vi "CRYFlatten Text Save.vi"(5 "Origin Text":string, 6 "error in":errorcluster, 7 "Type In":enum16{"Curves", "Values", "Results", "WFM"}(ring), 8 "Any Flatten Data":string, 9 "Path In":path) -> (0 "error out":errorcluster, 3 "Path Out":path)   [LabVIEW 2013]
uses:
  CRYSystem/Typedef Control/CRYData Cluster Array.ctl
  CRYSystem/Typedef Control/CRYData Cluster.ctl
  CRYSystem/Typedef Control/CRYWaveform Cluster Array.ctl
  CRYSystem/Typedef Control/CRYWaveform Cluster.ctl
  CRYSystem/Typedef Control/CRYResult Cluster Array.ctl
  CRYSystem/Typedef Control/CRYResult Cluster.ctl
panel:
  in  "Results":T1 {"Margin" format="%.2f"}
  in  "Waveforms":T3 {"Y dB ref" format="%.1f"; "Y axis" items=["Log", "Lin"]; "Y data" items=["dB", "Lin"]; "X data" items=["dB", "Lin"]}
  in  "Curves":T5 {"Z data" items=["dB", "Lin"]; "X data" items=["dB", "Lin"]; "Y data" items=["dB", "Lin"]; "Z dB ref" format="%.1f"; "Z axis" items=["Log", "Lin"]; "X dB ref" format="%.1f"; "X axis" items=["Log", "Lin"]; "Y axis" items=["Log", "Lin"]; "Y dB ref" format="%.1f"; "Curve"."z" format="%.2f"; "Curve"."y" format="%.2f"; "Curve"."x" format="%.2f"}
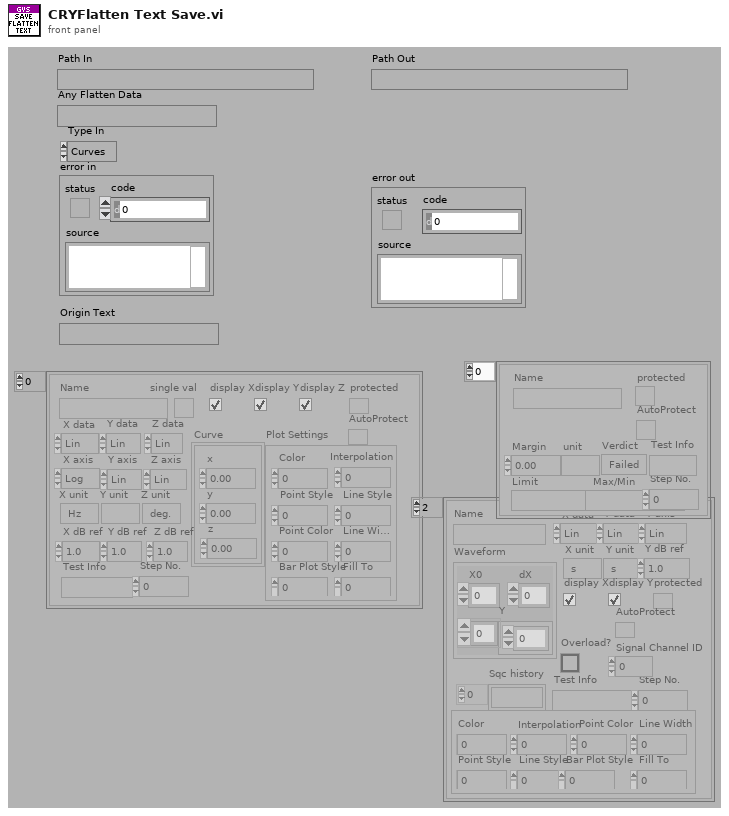
[diagram p1: front panel]
types:
  T1 = typedef "CRYResult Cluster Array.ctl" = T2[]
  T2 = typedef "CRYResult Cluster.ctl" = cluster{"Name":string, "Margin":dbl, "unit":string, "Verdict":bool, "Limit":string, "Max/Min":string, "protected":bool, "Step No.":i32, "Test Info":string, "AutoProtect":bool}
  T3 = typedef "CRYWaveform Cluster Array.ctl" = T4[]
  T4 = typedef "CRYWaveform Cluster.ctl" = cluster{"Waveform":cluster{"X0":dbl, "dX":dbl, "Y":sgl[]}, "X data":u16, "Y data":u16, "Y axis":u16, "X unit":string, "Y unit":string, "Y dB ref":dbl, "display Y":bool, "display X":bool, "Overload?":bool, "Test Info":string, "Step No.":i32, "Name":string, "protected":bool, "Sqc history":string[], "Signal Channel ID":i32, "Plot Settings":cluster{"Color":u32, "Interpolation":u8, "Point Style":u8, "Line Style":u8, "Point Color":u32, "Line Width":u8, "Bar Plot Style":u8, "Fill To":i16}, "AutoProtect":bool}
  T5 = typedef "CRYData Cluster Array.ctl" = T6[]
  T6 = typedef "CRYData Cluster.ctl" = cluster{"Name":string, "Curve":cluster{"x":dbl, "y":dbl, "z":dbl}[], "X data":u16, "Y data":u16, "Z data":u16, "X axis":u16, "Y axis":u16, "Z axis":u16, "X unit":string, "Y unit":string, "Z unit":string, "X dB ref":dbl, "Y dB ref":dbl, "Z dB ref":dbl, "single val":bool, "protected":bool, "display X":bool, "display Y":bool, "display Z":bool, "Test Info":string, "Step No.":i32, "Plot Settings":cluster{"Color":u32, "Interpolation":u8, "Point Style":u8, "Line Style":u8, "Point Color":u32, "Line Width":u8, "Bar Plot Style":u8, "Fill To":i16}, "AutoProtect":bool}
  T7 = enum16{"open", "replace", "create", "open or create", "replace or create", "replace or create with confirmation"}
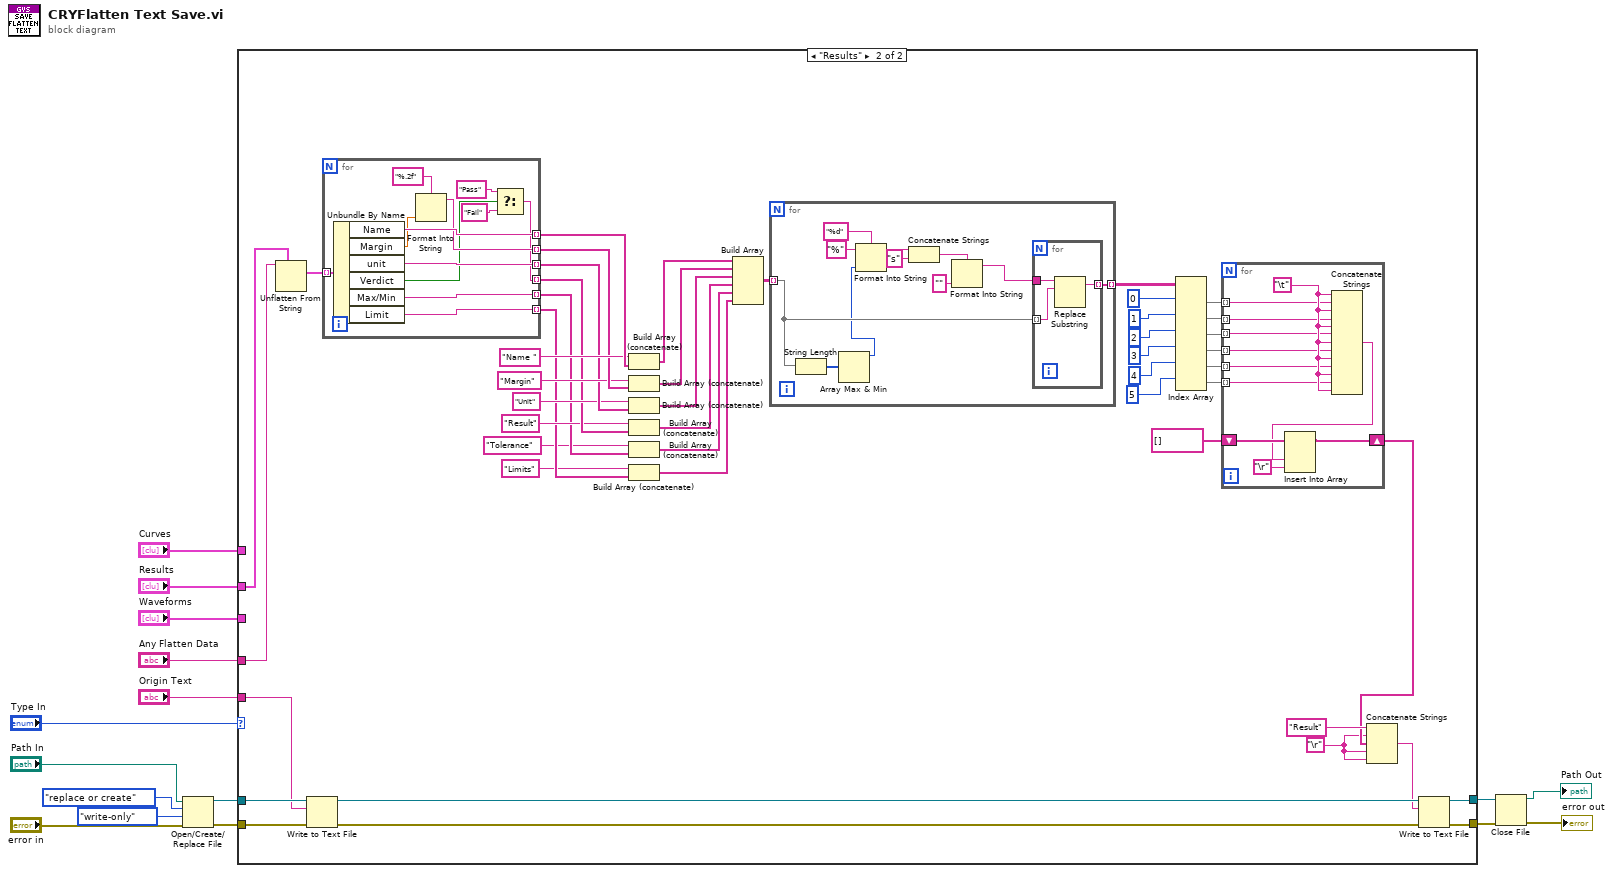
[diagram p0: block diagram]
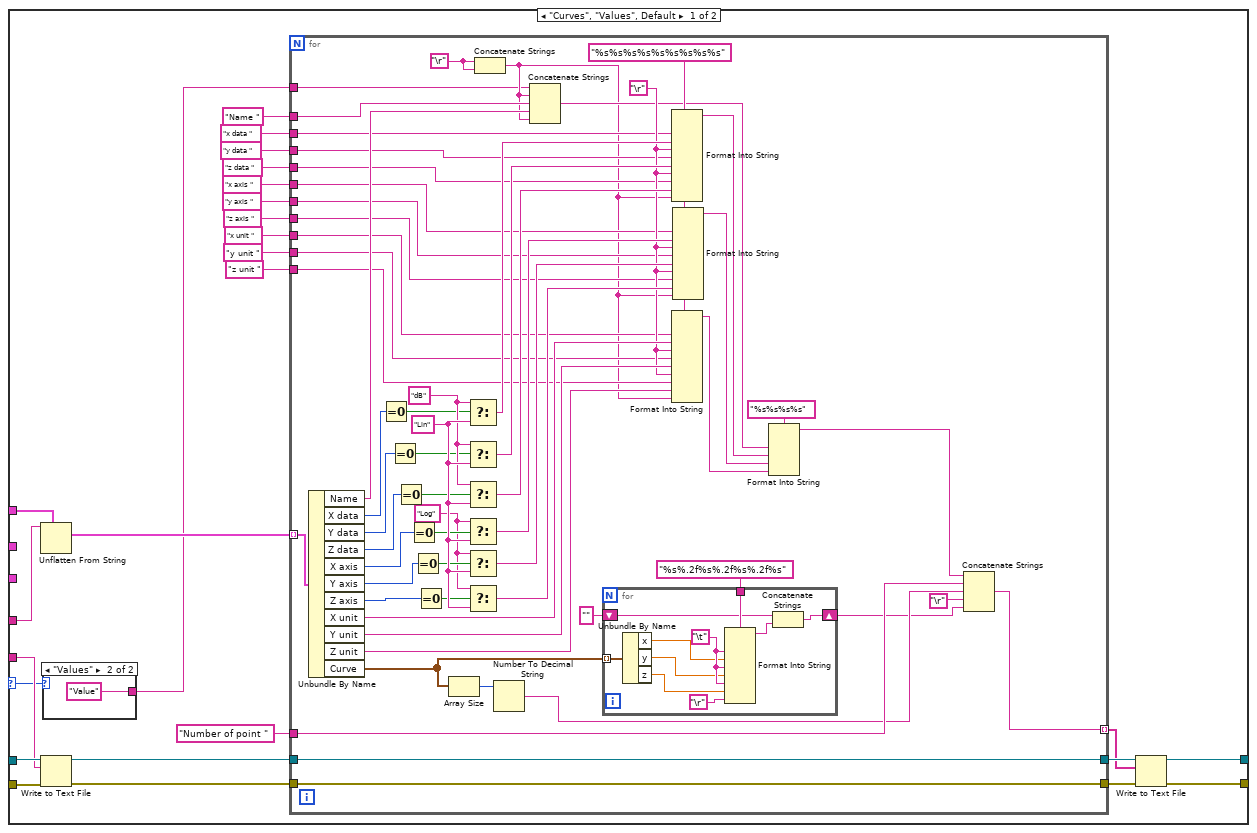
[diagram p2: hidden frame]
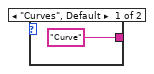
[diagram p3: hidden frame]
diagram:
  n1 = Open/Create/Replace File(file path (use dialog)="Path In", error in="error in", operation (0:open)=T7."replace or create", access (0:read/write)=enum16{"read/write", "read-only", "write-only"}."write-only") -> (refnum out=w7:refnum<file>, error out=w6:errorcluster)  [unwired: 3 out]
  n2 = case shown="\"Results\"" "Type In" {
    selector: "Type In" -> [w35 _]
    tunnel: "Any Flatten Data" -> [w41 w159]
    tunnel: [w21 w142] -> w4
    tunnel: "Curves" -> [w42 _]
    tunnel: "Results" -> [_ w158]
    tunnel: "Waveforms" -> [_ _]
    tunnel: w7 -> [w40 w141]
    tunnel: w6 -> [w38 w139]
    tunnel: [w23 w143] -> w5
    tunnel: "Origin Text" -> [w36 w117]
    frame "Curves", "Values", Default {
      n3 = Unflatten From String(type=w42, binary string=w41) -> (value=w25:T5)  [unwired: 1 in, 4 out]
      n4 = Write to Text File(file (use dialog)=w40, text=w36, error in=w38) -> (refnum out=w39:refnum<file>, error out=w37:errorcluster)  [unwired: 1 in, 1 out]
      n5 = case shown="\"Values\"" w35 {
        tunnel: ["Curve" "Value"] -> w18
        frame "Curves", Default {
        }
        frame "Values" {
        }
      }
      n6 = for {
        tunnel: w39 -> [w59]
        tunnel: [w59] -> w24
        tunnel: [w58] -> w22
        tunnel: w37 -> [w58]
        tunnel: w25 -> [w102] mode=indexing
        tunnel: "x data " -> [w70]
        tunnel: "y data " -> [w69]
        tunnel: "z data " -> [w68]
        tunnel: "x axis " -> [w67]
        tunnel: "y axis " -> [w66]
        tunnel: "z axis " -> [w65]
        tunnel: "x unit " -> [w64]
        tunnel: "y unit " -> [w63]
        tunnel: "z unit " -> [w62]
        tunnel: "Name " -> [w55]
        tunnel: [w56] -> w19 mode=indexing
        tunnel: w18 -> [w52]
        tunnel: "Number of point " -> [w51]
        w79 = "%s%s%s%s%s%s%s%s%s" ("format string")
        w86 = "Log"
        w100 = "Lin"
        w99 = "dB"
        w76 = "\r"
        w54 = "\r"
        n7 = Unbundle By Name(w102) -> ("Name"=w101:string, "X data"=w87:u16, "Y data"=w88:u16, "Z data"=w89:u16, "X axis"=w90:u16, "Y axis"=w91:u16, "Z axis"=w92:u16, "X unit"=w78:string, "Y unit"=w77:string, "Z unit"=w75:string, "Curve"=w50:cluster{"x":dbl, "y":dbl, "z":dbl}[])
        n8 = Equal To 0?(x=w87) -> (x = 0?=w93:bool)
        n9 = Equal To 0?(x=w88) -> (x = 0?=w94:bool)
        n10 = Equal To 0?(x=w89) -> (x = 0?=w95:bool)
        n11 = Equal To 0?(x=w90) -> (x = 0?=w96:bool)
        n12 = Equal To 0?(x=w91) -> (x = 0?=w97:bool)
        n13 = Equal To 0?(x=w92) -> (x = 0?=w98:bool)
        n14 = Array Size(array=w50) -> (size(s)=w49:i32)
        n15 = Select(t=w99, s=w93, f=w100) -> (s? t:f=w85:string)
        n16 = Select(t=w99, s=w94, f=w100) -> (s? t:f=w84:string)
        n17 = Select(t=w99, s=w95, f=w100) -> (s? t:f=w83:string)
        n18 = Select(t=w86, s=w96, f=w100) -> (s? t:f=w82:string)
        n19 = Select(t=w86, s=w97, f=w100) -> (s? t:f=w81:string)
        n20 = Select(t=w86, s=w98, f=w100) -> (s? t:f=w80:string)
        n21 = Concatenate Strings(w54, w54) -> (w53:string)
        n22 = Number To Decimal String(number=w49) -> (decimal integer string=w47:string)  [unwired: 1 in]
        n23 = Concatenate Strings(w52, w53, w55, w101, w53) -> (w57:string)
        n24 = for {
          tunnel: w50 -> [w112] mode=indexing
          tunnel: "%s%.2f%s%.2f%s%.2f%s" ("format string") -> [w109]
          shift-right: [w103] -> w45
          shift-left: "" -> [w105]
          w111 = "\t"
          n25 = Unbundle By Name(w112) -> ("x"=w108:dbl, "y"=w107:dbl, "z"=w106:dbl)
          n26 = Format Into String(format string=w109, w111, w108, w111, w107, w111, w106, "\r") -> (resulting string=w104:string)  [unwired: 2 in, 1 out]
          n27 = Concatenate Strings(w105, w104) -> (w103:string)
        }
        n28 = Format Into String(format string=w79, w70, w85, w76, w69, w84, w76, w68, w83, w53) -> (resulting string=w74:string)  [unwired: 2 in, 1 out]
        n29 = Format Into String(format string=w79, w64, w78, w76, w63, w77, w76, w62, w75, w53) -> (resulting string=w72:string)  [unwired: 2 in, 1 out]
        n30 = Format Into String(format string=w79, w67, w82, w76, w66, w81, w76, w65, w80, w53) -> (resulting string=w73:string)  [unwired: 2 in, 1 out]
        n31 = Format Into String(format string="%s%s%s%s", w57, w74, w73, w72) -> (resulting string=w46:string)  [unwired: 2 in, 1 out]
        n32 = Concatenate Strings(w46, w51, w47, "\r", w45) -> (w56:string)
      }
      n33 = Write to Text File(file (use dialog)=w24, text=w19, error in=w22) -> (refnum out=w23:refnum<file>, error out=w21:errorcluster)  [unwired: 1 in, 1 out]
    }
    frame "Results" {
      w114 = "\r"
      n34 = Unflatten From String(type=w158, binary string=w159) -> (value=w157:T1)  [unwired: 1 in, 4 out]
      n35 = Write to Text File(file (use dialog)=w141, text=w117, error in=w139) -> (refnum out=w140:refnum<file>, error out=w138:errorcluster)  [unwired: 1 in, 1 out]
      n36 = for {
        tunnel: w157 -> [w196] mode=indexing
        tunnel: [w195] -> w156 mode=indexing
        tunnel: [w194] -> w152 mode=indexing
        tunnel: [w193] -> w148 mode=indexing
        tunnel: [w192] -> w147 mode=indexing
        tunnel: [w189] -> w154 mode=indexing
        tunnel: [w185] -> w150 mode=indexing
        n37 = Unbundle By Name(w196) -> ("Name"=w195:string, "Margin"=w190:dbl, "unit"=w194:string, "Verdict"=w188:bool, "Max/Min"=w193:string, "Limit"=w192:string)
        n38 = Format Into String(format string="%.2f", w190) -> (resulting string=w189:string)  [unwired: 2 in, 1 out]
        n39 = Select(t="Pass", s=w188, f="Fail") -> (s? t:f=w185:string)
      }
      n40 = Build Array (concatenate)("Name ", w156) -> (w137:string[])
      n41 = Build Array (concatenate)("Margin", w154) -> (w136:string[])
      n42 = Build Array (concatenate)("Unit", w152) -> (w135:string[])
      n43 = Build Array (concatenate)("Result", w150) -> (w134:string[])
      n44 = Build Array (concatenate)("Tolerance", w148) -> (w133:string[])
      n45 = Build Array (concatenate)("Limits", w147) -> (w132:string[])
      n46 = Build Array(w137, w136, w135, w134, w133, w132) -> (w131:string[][])
      n47 = for {
        tunnel: w131 -> [w163] mode=indexing
        tunnel: [w162] -> w130 mode=indexing
        n48 = String Length(string=w163) -> (length=w161:i32[])
        n49 = Array Max & Min(array=w161) -> (max value=w160:i32)  [unwired: 3 out]
        n50 = Format Into String(format string="%d", initial string="%", w160) -> (resulting string=w167:string)  [unwired: 1 in, 1 out]
        n51 = Concatenate Strings(w167, "s" ("string")) -> (w165:string)
        n52 = Format Into String(format string=w165, "" ("input 1")) -> (resulting string=w164:string)  [unwired: 2 in, 1 out]
        n53 = for {
          tunnel: w164 -> [w173]
          tunnel: w163 -> [w172] mode=indexing
          tunnel: [w171] -> w162 mode=indexing
          n54 = Replace Substring(4:w172, 5:w173) -> (1:w171:string)  [unwired: 3 out]
        }
      }
      n55 = Index Array(array=w130, index (row) #1=0 ("index (row)"), index (row) #2=1 ("index (row)"), index (row) #3=2 ("index (row)"), index (row) #4=3 ("index (row)"), index (row) #5=4 ("index (row)"), index (row) #6=5 ("index (row)")) -> (element #1=w129:string[], element #2=w128:string[], element #3=w127:string[], element #4=w126:string[], element #5=w125:string[], element #6=w124:string[])  [unwired: 6 in]
      n56 = for {
        shift-right: [w183] -> w115
        shift-left: string[] [] -> [w184]
        tunnel: w129 -> [w180] mode=indexing
        tunnel: w128 -> [w179] mode=indexing
        tunnel: w127 -> [w178] mode=indexing
        tunnel: w126 -> [w177] mode=indexing
        tunnel: w125 -> [w176] mode=indexing
        tunnel: w124 -> [w175] mode=indexing
        w181 = "\t"
        n57 = Concatenate Strings(w181, w180, w181, w179, w181, w178, w181, w177, w181, w176, w181, w175, w181) -> (w182:string)
        n58 = Insert Into Array(array=w184, new element #1=w182, new element #2="\r") -> (w183:string[])  [unwired: 1 in]
      }
      n59 = Concatenate Strings("Result" ("match + rest of string"), w114, w115, w114, w114) -> (w113:string)
      n60 = Write to Text File(file (use dialog)=w140, text=w113, error in=w138) -> (refnum out=w143:refnum<file>, error out=w142:errorcluster)  [unwired: 1 in, 1 out]
    }
  }
  n61 = Close File(refnum=w5, error in=w4) -> (path=→"Path Out":path, error out=→"error out":errorcluster)
